vi "Start Channel.vi"(6 "Filter":T1 {"Config"."End" format="%x"; "Config"."Start" format="%x"}, 8 "error in (no error)":errorcluster, 9 "ChannelType":enum16{"Device", "Ch0", "Ch1"}(ring), 10 "Param":T2={"Terminal"=0, "Param"={"abitbaud"=500000, "dbitbaud"=500000, "CustomBaud"=FALSE, "CustomBd"="", "Mode"=0, "Standard"=0}} {"Param"."Standard" items=["CANFD ISO", "CANFD BOSCH"]; "Param"."dbitbaud" items=["5Mbps"=5000000, "4Mbps"=4000000, "2Mbps"=2000000, "1Mbps"=1000000, "800kbps"=800000, "500kbps"=500000, "250kbps"=250000, "125kbps"=125000, "100kbps"=100000]; "Param"."abitbaud" items=["1Mbps"=1000000, "800kbps"=800000, "500kbps"=500000, "250kbps"=250000, "125kbps"=125000, "100kbps"=100000, "50kbps"=50000]; "Param"."Mode" items=["正常", "只听"]; "Terminal" items=["禁用", "启用"]}, 11 "DevState":T3={"Type"=41, "Index"=0, "DeviceOpen"=FALSE, "Ch0Start"=FALSE, "Ch1Start"=FALSE} {"Index" items=["0", "1", "2", "3", "4", "5", "6", "7", "8"]; "Type" items=["USBCANFD-200U"=41, "USBCANFD-100U"=42]}) -> (0 "error out":errorcluster, 3 "DevState out":T3={"Type"=41, "Index"=0, "DeviceOpen"=FALSE, "Ch0Start"=FALSE, "Ch1Start"=FALSE} {"Index" items=["0", "1", "2", "3", "4", "5", "6", "7", "8"]; "Type" items=["USBCANFD-200U"=41, "USBCANFD-100U"=42]})   [LabVIEW 2011, in "CAN FD.lvlib"]
uses:
  CAN FD.lvlib
  SubVI/zlgcan.lvlib
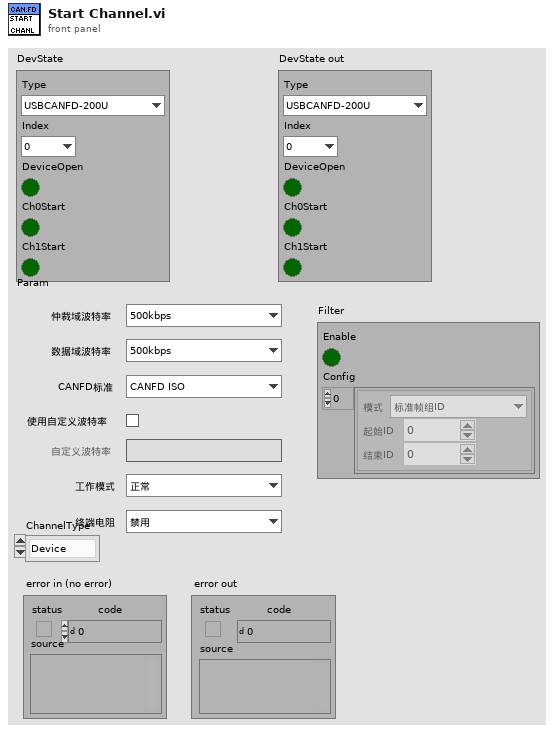
[diagram p1: front panel]
types:
  T1 = cluster{"Enable":bool, "Config":cluster{"Mode":enum16{"标准帧组ID", "标准帧明确ID", "扩展帧组ID", "扩展帧明确ID"}, "Start":u32, "End":u32}[]}
  T2 = cluster{"Terminal":u32, "Param":cluster{"abitbaud":u32, "dbitbaud":u32, "CustomBaud":bool, "CustomBd":string, "Mode":u8, "Standard":u32}}
  T3 = cluster{"Type":u32, "Index":u32, "DeviceOpen":bool, "Ch0Start":bool, "Ch1Start":bool}
  T4 = cluster{"abitbaud":u32, "dbitbaud":u32, "CustomBaud":bool, "CustomBd":string, "Mode":u8, "Standard":u32}
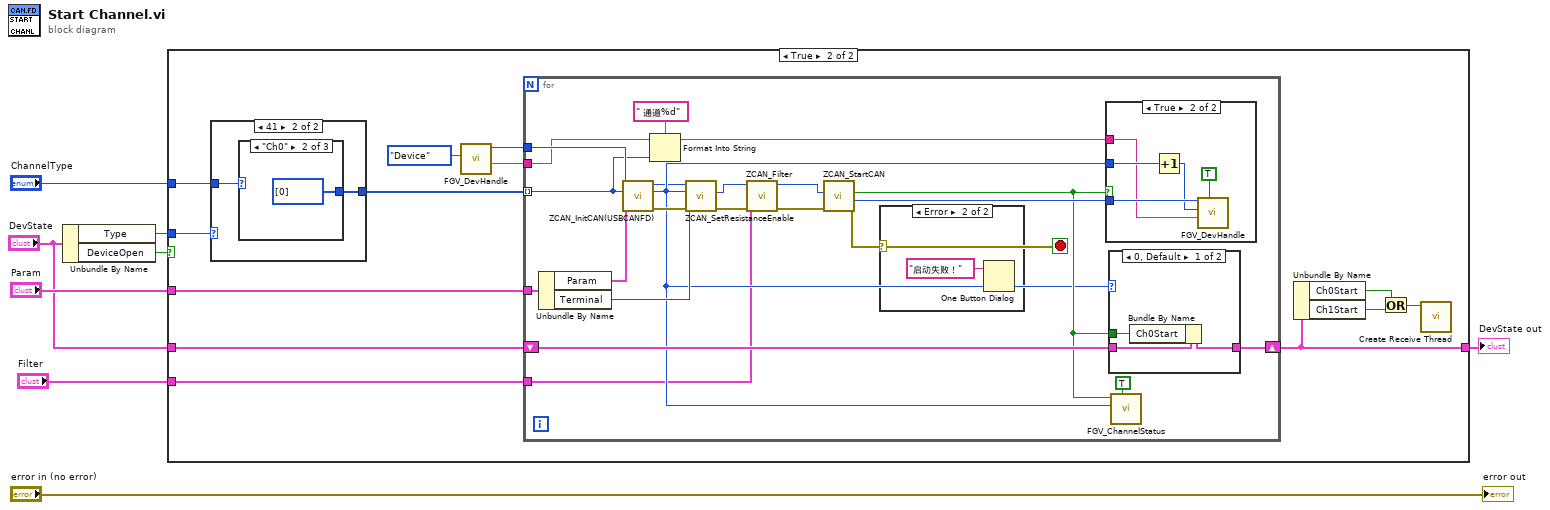
[diagram p0: block diagram]
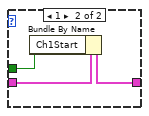
[diagram p4: hidden frame]
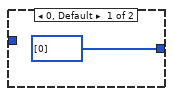
[diagram p6: hidden frame]
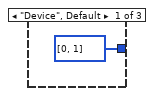
[diagram p7: hidden frame]
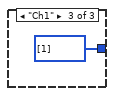
[diagram p8: hidden frame]
diagram:
  n1 = Unbundle By Name("DevState") -> ("Type"=w7:u32, "DeviceOpen"=w5:bool)
  n2 = case shown="True" w5 {
    tunnel: w7 -> [_ w22]
    tunnel: "ChannelType" -> [_ w21]
    tunnel: "Param" -> [_ w19]
    tunnel: "DevState" -> [w9 w16]
    tunnel: [w9 w15] -> w2
    tunnel: "Filter" -> [_ w10]
    frame False {
    }
    frame True {
      n3 = case shown="41" w22 {
        tunnel: w21 -> [_ w57]
        tunnel: [i32[] [0] w56] -> w20
        frame 0, Default {
        }
        frame 41 {
          n4 = case shown="\"Ch0\"" w57 {
            tunnel: [i32[] [0, 1] i32[] [0] i32[] [1]] -> w56
            frame "Device", Default {
            }
            frame "Ch0" {
            }
            frame "Ch1" {
            }
          }
        }
      }
      n5 = call "FGV_DevHandle.vi"("Type"=enum16{"Device", "Ch0", "Ch1"}."Device") -> ("Name out"=w11:string, "handle out"=w17:u32)  [unwired: 8 in, 1 out]
      n6 = for {
        tunnel: w20 -> [w31] mode=indexing
        tunnel: w19 -> [w40]
        tunnel: w17 -> [w38]
        shift-right: [w35] -> w15
        shift-left: w16 -> [w36]
        tunnel: w11 -> [w30]
        tunnel: w10 -> [w27]
        stop <- w25 stop-if-true
        n7 = Unbundle By Name(w40) -> ("Param"=w42:T4, "Terminal"=w41:u32)
        n8 = call "ZCAN_InitCAN(USBCANFD).vi"("device_hande"=w38, "can_index"=w31, "ZCAN_InitCAN_Setting_USBCANFD"=w42) -> ("can_index_handle"=w28:u32, "error out"=w39:errorcluster)  [unwired: 11 in]
        n9 = Format Into String(format string=" 通道%d" ("格式字符串"), initial string=w30, w31) -> (resulting string=w29:string)  [unwired: 1 in, 1 out]
        n10 = call "ZCAN_SetResistanceEnable.vi"("error in (no error)"=w39, "enable"=w41, "can_index"=w31, "can_index_handle"=w28) -> ("error out"=w24:errorcluster, "can_index_handle(out)"=w26:u32)  [unwired: 6 in]
        n11 = call "ZCAN_Filter.vi"("error in (no error)"=w24, "Filter"=w27, "channel_handle"=w26) -> ("error out"=w23:errorcluster)  [unwired: 7 in]
        n12 = call "ZCAN_StartCAN.vi"("error in (no error)"=w23, "can_index_handle"=w26) -> ("error out"=w25:errorcluster, "can_index_handle(out)"=w37:u32, "startcan_success?"=w34:bool)  [unwired: 7 in]
        n13 = case shown="Error" w25 {
          frame No Error {
          }
          frame Error {
            n14 = One Button Dialog(message="启动失败！" ("消息")) -> ()  [unwired: 1 in, 1 out]
          }
        }
        n15 = case shown="True" w34 {
          tunnel: w37 -> [_ w54]
          tunnel: w31 -> [_ w53]
          tunnel: w29 -> [_ w50]
          frame False {
          }
          frame True {
            n16 = Increment(x=w53) -> (x+1=w52:i32)
            n17 = call "FGV_DevHandle.vi"("Set"=TRUE, "Name"=w50, "Type"=w52, "handle"=w54) -> ()  [unwired: 5 in, 3 out]
          }
        }
        n18 = case shown="0, Default" w31 {
          tunnel: w34 -> [w45 w48]
          tunnel: w36 -> [w46 w49]
          tunnel: [w44 w47] -> w35
          frame 0, Default {
            n19 = Bundle By Name(cluster=w46, "Ch0Start"=w45) -> (w44:T3)
          }
          frame 1 {
            n20 = Bundle By Name(cluster=w49, "Ch1Start"=w48) -> (w47:T3)
          }
        }
        n21 = call "FGV_ChannelStatus.vi"("Set"=TRUE, "Index"=w31, "Start"=w34) -> ()  [unwired: 7 in, 2 out]
      }
      n22 = Unbundle By Name(w15) -> ("Ch0Start"=w13:bool, "Ch1Start"=w14:bool)
      n23 = Or(x=w13, y=w14) -> (x .or. y?=w12:bool)
      n24 = call "Create Receive Thread.vi"("OpenStatus"=w12) -> ()  [unwired: 11 in]
    }
  }
  "DevState out" <- w2
  "error out" <- "error in (no error)"
